vi "Handle Errors.vi"() -> (1 "General":bool, 2 "PAS":bool, 3 "CRD":bool)   [LabVIEW 2015, in "cPAS Facade.lvclass"]
uses:
  cPAS Facade.lvclass
  Reusable/Error Logging/Error Logger.lvclass
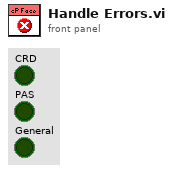
[diagram p1: front panel]
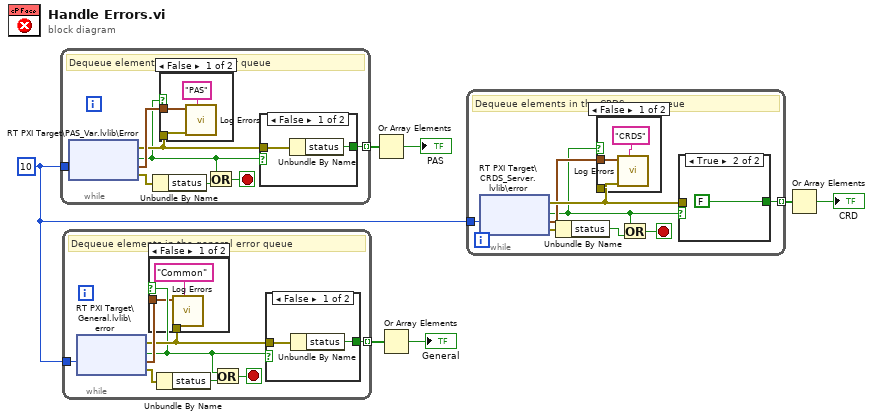
[diagram p0: block diagram]
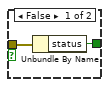
[diagram p3: hidden frame]
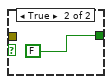
[diagram p5: hidden frame]
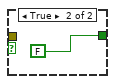
[diagram p7: hidden frame]
diagram:
  w5 = 10 ("ms timeout (0)")
  n1 = while "Dequeue elements in the PAS error queue" {
    tunnel: [w15] -> w7 mode=indexing
    tunnel: w5 -> [w13]
    stop <- w12 stop-if-true
    # "Dequeue elements in the PAS error queue"
    n2 = shared-variable "RT PXI Target\\PAS_Var.lvlib\\Error"(w13) -> (w9:errorcluster, error out=w10:errorcluster, w11:timestamp, w8:bool)  [unwired: 1 in]
    n3 = Unbundle By Name(w10) -> ("status"=w14:bool)
    n4 = case shown="False" w8 {
      tunnel: w11 -> [w17 _]
      tunnel: w9 -> [w16 _]
      frame False {
        n5 = call "Log Errors.vi"("System"="PAS", "error in"=w16, "Time Stamp"=w17) -> ()  [unwired: 8 in, 1 out]
      }
      frame True {
      }
    }
    n6 = Or(x=w8, y=w14) -> (x .or. y?=w12:bool)
    n7 = case shown="False" w8 {
      tunnel: [w20 FALSE ("status")] -> w15
      tunnel: w9 -> [w19 _]
      frame False {
        n8 = Unbundle By Name(w19) -> ("status"=w20:bool)
      }
      frame True {
      }
    }
  }
  n9 = while "Dequeue elements in the PAS error queue" {
    tunnel: [w29] -> w6 mode=indexing
    tunnel: w5 -> [w26]
    stop <- w25 stop-if-true
    # "Dequeue elements in the general error queue"
    n10 = shared-variable "RT PXI Target\\General.lvlib\\error"(w26) -> (w23:errorcluster, error out=w27:errorcluster, w24:timestamp, w22:bool)  [unwired: 1 in]
    n11 = case shown="False" w22 {
      tunnel: w24 -> [w31 _]
      tunnel: w23 -> [w30 _]
      frame False {
        n12 = call "Log Errors.vi"("System"="Common", "error in"=w30, "Time Stamp"=w31) -> ()  [unwired: 8 in, 1 out]
      }
      frame True {
      }
    }
    n13 = Unbundle By Name(w27) -> ("status"=w28:bool)
    n14 = Or(x=w22, y=w28) -> (x .or. y?=w25:bool)
    n15 = case shown="False" w22 {
      tunnel: [w34 FALSE ("status")] -> w29
      tunnel: w23 -> [w33 _]
      frame False {
        n16 = Unbundle By Name(w33) -> ("status"=w34:bool)
      }
      frame True {
      }
    }
  }
  n17 = Or Array Elements(Boolean array=w7) -> (logical OR=→"PAS":bool)
  n18 = Or Array Elements(Boolean array=w6) -> (logical OR=→"General":bool)
  n19 = while "Dequeue elements in the PAS error queue" {
    tunnel: [w43] -> w4 mode=indexing
    tunnel: w5 -> [w40]
    stop <- w39 stop-if-true
    # "Dequeue elements in the CRDS error queue"
    n20 = shared-variable "RT PXI Target\\CRDS_Server.lvlib\\error"(w40) -> (w38:errorcluster, error out=w41:errorcluster, w37:timestamp, w36:bool)  [unwired: 1 in]
    n21 = Unbundle By Name(w41) -> ("status"=w42:bool)
    n22 = case shown="False" w36 {
      tunnel: w38 -> [w45 _]
      tunnel: w37 -> [w44 _]
      frame False {
        n23 = call "Log Errors.vi"("System"="CRDS", "error in"=w45, "Time Stamp"=w44) -> ()  [unwired: 8 in, 1 out]
      }
      frame True {
      }
    }
    n24 = Or(x=w36, y=w42) -> (x .or. y?=w39:bool)
    n25 = case shown="True" w36 {
      tunnel: [w48 FALSE ("status")] -> w43
      tunnel: w38 -> [w47 _]
      frame False {
        n26 = Unbundle By Name(w47) -> ("status"=w48:bool)
      }
      frame True {
      }
    }
  }
  n27 = Or Array Elements(Boolean array=w4) -> (logical OR=→"CRD":bool)
